vi "test Deployment With Configuration.vi"(8 "error in":errorcluster, 11 "TestCase in":refnum<class "Deployment.lvclass">) -> (0 "error out":errorcluster, 3 "TestCase out":refnum<class "Deployment.lvclass">)   [LabVIEW 2020, in "Deployment.lvclass"]
uses:
  Deployment.lvclass
  Shared/1553 Channel.ctl
  Shared/Terminal Name and Address.ctl
  Shared/Address.ctl
  Shared/Message Definition.ctl
  Shared/Message Type.ctl
  Shared/Terminal Endpoint.ctl
  Shared/Parameter Definition.ctl
  Deployment.lvclass/Deployment.ctl
  315b1c3a-44c8-49e8-b756-01f865c29b4a.vi
  <vilib>/addons/_JKI Toolkits/VI Tester/TestCase.llb/TestCase.lvclass
  niveristand-custom-device-testing-tools/VeriStandTestUtilities/VeriStandTestUtilities.lvlib
  Scripting/Ballard MIL-STD-1553 Scripting.lvlib
  C:/Program Files (x86)/National Instruments/LabVIEW 2020/vi.lib/addons/_JKI Toolkits/VI Tester/TestCase.llb/TestCase.lvclass
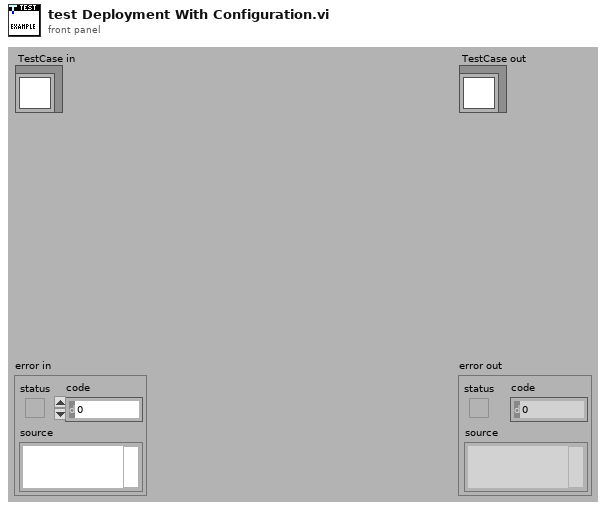
[diagram p1: front panel]
types:
  T1 = typedef "1553 Channel.ctl" = cluster{"HW channel":u16, "terminals":T2[], "messages":T4[], "acyclic frame names":string[]}
  T2 = typedef "Terminal Name and Address.ctl" = cluster{"name":string, "terminal address":T3}
  T3 = typedef "Address.ctl" = u16
  T4 = typedef "Message Definition.ctl" = cluster{"name":string, "message type":T5, "endpoint Rx":T6, "endpoint Tx":T6, "mode code":u16, "number of words":u16, "parameters":cluster{"name":string, "default value":dbl, "unit":string, "parameter definition":T7}[], "create timestamp channel":bool}
  T5 = typedef "Message Type.ctl" = string
  T6 = typedef "Terminal Endpoint.ctl" = cluster{"terminal address":T3, "subaddress":T3}
  T7 = typedef "Parameter Definition.ctl" = cluster{"start index":i32, "size (bits)":i32, "encoding":enum16{"BNR", "BCD", "Discrete"}, "signed":bool, "multiplier":dbl, "offset":dbl}
  T8 = typedef "Custom Device API.lvlib/Custom Device Item Ref.ctl" = u64
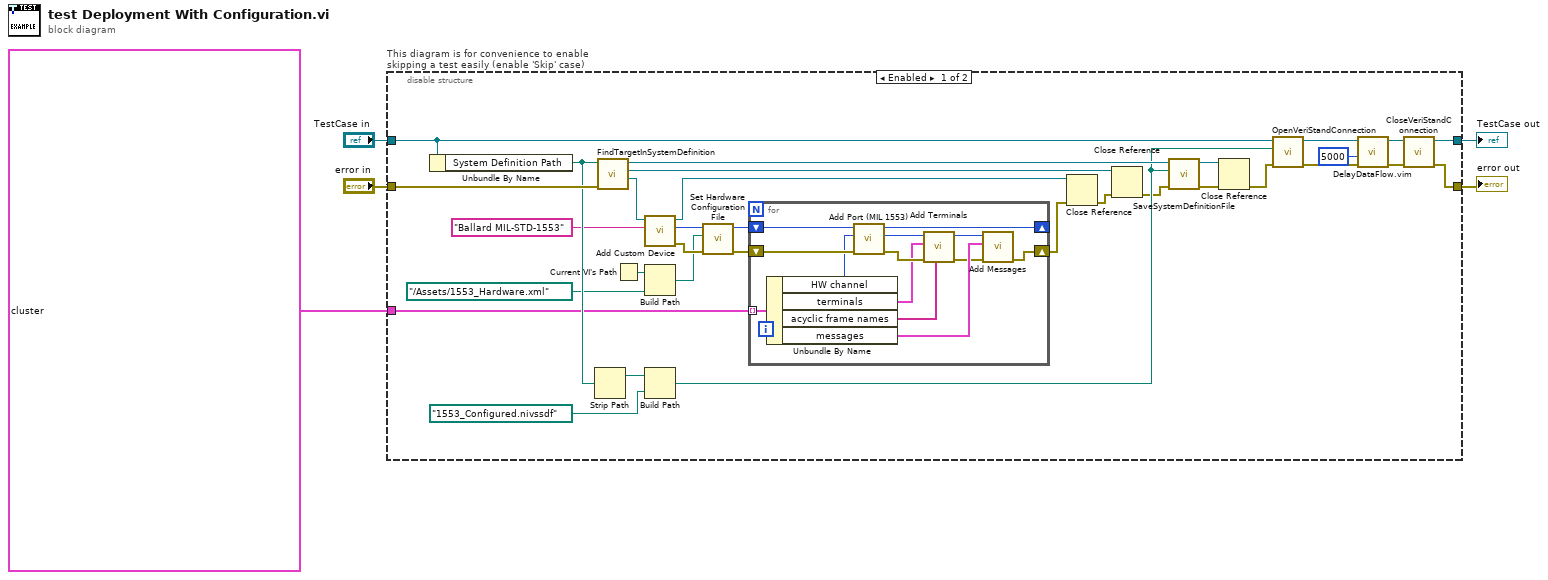
[diagram p0: block diagram]
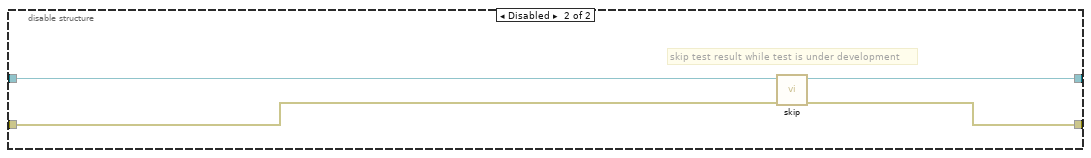
[diagram p2: hidden frame]
diagram:
  n1 = disable-structure "This diagram is for convenience to enable skipping a test easily (enable 'Skip' case)" shown="Enabled" {
    disable-tunnel: "TestCase in" -> [w30 w53]
    disable-tunnel: [w31 w51] -> w2
    disable-tunnel: [w33 w52] -> w4
    disable-tunnel: "error in" -> [w29 w50]
    disable-tunnel: T1[] [{"HW channel"=0, "terminals"=[{"name"="Bus Controller", "terminal address"=0}, {"name"="Remote Terminal 1", "terminal address"=1}, {"name"="Remote Terminal 15", "terminal address"=15}, {"name"="Remote Terminal 21", "terminal address"=21}, {"name"="Remote Terminal 31 (Broadcast)", "terminal address"=31}], "messages"=[{"name"="BC to RT 1.2", "message type"="BC to RT", "endpoint Rx"={"terminal address"=1, "subaddress"=2}, "endpoint Tx"={"terminal address"=0, "subaddress"=0}, "mode code"=0, "number of words"=3, "parameters"=[], "create timestamp channel"=FALSE}, {"name"="RT 31.15 to RT 21.21", "message type"="RT to RT", "endpoint Rx"={"terminal address"=31, "subaddress"=21}, "endpoint Tx"={"terminal address"=15, "subaddress"=21}, "mode code"=0, "number of words"=11, "parameters"=[], "create timestamp channel"=FALSE}, {"name"="BC to RT 3.0", "message type"="BC to RT", "endpoint Rx"={"terminal address"=1, "subaddress"=3}, "endpoint Tx"={"terminal address"=0, "subaddress"=0}, "mode code"=0, "number of words"=4, "parameters"=[], "create timestamp channel"=FALSE}, {"name"="RT 1.5 to BC", "message type"="RT to BC", "endpoint Rx"={"terminal address"=0, "subaddress"=0}, "endpoint Tx"={"terminal address"=1, "subaddress"=5}, "mode code"=0, "number of words"=6, "parameters"=[], "create timestamp channel"=FALSE}, {"name"="RT 1.6 to BC", "message type"="RT to BC", "endpoint Rx"={"terminal address"=0, "subaddress"=0}, "endpoint Tx"={"terminal address"=1, "subaddress"=6}, "mode code"=0, "number of words"=2, "parameters"=[], "create timestamp channel"=FALSE}, {"name"="RT 15.20 to RT 1.20", "message type"="RT to RT", "endpoint Rx"={"terminal address"=15, "subaddress"=20}, "endpoint Tx"={"terminal address"=1, "subaddress"=20}, "mode code"=0, "number of words"=4, "parameters"=[], "create timestamp channel"=FALSE}, {"name"="MC 16", "message type"="MC", "endpoint Rx"={"terminal address"=0, "subaddress"=0}, "endpoint Tx"={"terminal address"=1, "subaddress"=31}, "mode code"=16, "number of words"=1, "parameters"=[], "create timestamp channel"=FALSE}, {"name"="MC 17", "message type"="MC", "endpoint Rx"={"terminal address"=1, "subaddress"=31}, "endpoint Tx"={"terminal address"=0, "subaddress"=0}, "mode code"=17, "number of words"=1, "parameters"=[], "create timestamp channel"=FALSE}, {"name"="BC to RT 31.28", "message type"="BC to RT", "endpoint Rx"={"terminal address"=31, "subaddress"=28}, "endpoint Tx"={"terminal address"=0, "subaddress"=0}, "mode code"=0, "number of words"=6, "parameters"=[], "create timestamp channel"=FALSE}, {"name"="MC 1", "message type"="MC", "endpoint Rx"={"terminal address"=31, "subaddress"=31}, "endpoint Tx"={"terminal address"=0, "subaddress"=0}, "mode code"=1, "number of words"=0, "parameters"=[], "create timestamp channel"=FALSE}], "acyclic frame names"=["acyclicFrame ID56"]}] -> [w13 _]
    frame Enabled {
      n2 = Unbundle By Name(w30) -> ("System Definition Path"=w27:path)
      n3 = Strip Path(path=w27) -> (stripped path=w26:path)  [unwired: 1 out]
      n4 = call "FindTargetInSystemDefinition.vi"("error in"=w29, "system definition path"=w27) -> ("Target"=w24:refnum<k24>, "Root"=w19:refnum<k24>, "System Definition"=w28:refnum<k24>)  [unwired: 6 in, 1 out]
      n5 = Current VI's Path() -> (path=w8:path)
      n6 = call "Add Custom Device.vi"("name"="Ballard MIL-STD-1553", "target in"=w24) -> ("error out"=w11:errorcluster, "Ballard MIL-STD-1553 custom device"=w12:T8, "target out"=w17:refnum<k24>)  [unwired: 7 in]
      n7 = Build Path(base path=w8, name or relative path=path "../Assets/1553_Hardware.xml") -> (appended path=w6:path)
      n8 = Build Path(base path=w26, name or relative path=path "1553_Configured.nivssdf") -> (appended path=w20:path)
      n9 = call "Set Hardware Configuration File.vi"("error in"=w11, "hardware configuration file path"=w6, "Ballard MIL-STD 1553 custom device in"=w12) -> ("error out"=w10:errorcluster, "Ballard MIL-STD 1553 custom device out"=w9:T8)  [unwired: 7 in]
      n10 = for {
        shift-right: [w45] -> _
        shift-left: w9 -> [w48]
        tunnel: w13 -> [w49] mode=indexing
        shift-right: [w43] -> w15
        shift-left: w10 -> [w47]
        n11 = Unbundle By Name(w49) -> ("HW channel"=w46:u16, "terminals"=w38:T2[], "acyclic frame names"=w37:string[], "messages"=w44:T4[])
        n12 = call "Add Port (MIL 1553).vi"("error in"=w47, "port number"=w46, "Ballard MIL-STD 1553 custom device in"=w48) -> ("error out"=w41:errorcluster, "port"=w42:T8, "Ballard MIL-STD 1553 custom device out"=w45:T8)  [unwired: 6 in]
        n13 = call "Add Terminals.vi"("acyclic frame names"=w37, "error in"=w41, "terminals"=w38, "port in"=w42) -> ("error out"=w39:errorcluster, "port out"=w40:T8)  [unwired: 6 in]
        n14 = call "Add Messages.vi"("error in"=w39, "messages"=w44, "port in"=w40) -> ("error out"=w43:errorcluster)  [unwired: 7 in, 1 out]
      }
      n15 = Close Reference(reference=w17, error in (no error)=w15) -> (error out=w16:errorcluster)
      n16 = Close Reference(reference=w19, error in (no error)=w16) -> (error out=w18:errorcluster)
      n17 = call "SaveSystemDefinitionFile.vi"("error in (no error)"=w18, "System Definition File in"=w20, "System Definition Reference in"=w28) -> ("error out"=w22:errorcluster, "System Definition Reference out"=w23:refnum<k24>)  [unwired: 7 in]
      n18 = Close Reference(reference=w23, error in (no error)=w22) -> (error out=w21:errorcluster)
      n19 = call-dynamic "OpenVeriStandConnection.vi"("error in (no error)"=w21, "System Definition File"=w20, "VeriStand Test Case in"=w30) -> ("error out"=w36:errorcluster, "VeriStand Test Case out"=w32:refnum<class "Deployment.lvclass">)  [unwired: 6 in, 1 out]
      n20 = call "DelayDataFlow.vim"("value in"=w36, "milliseconds to wait"=u32 5000) -> ("value out"=w34:errorcluster)  [unwired: 2 in, 1 out]
      n21 = call-dynamic "CloseVeriStandConnection.vi"("error in (no error)"=w34, "VeriStand Test Case in"=w32) -> ("error out"=w33:errorcluster, "VeriStand Test Case out"=w31:refnum<class "Deployment.lvclass">)  [unwired: 8 in]
    }
    frame Disabled {
      # "skip test result while test is under development"
      n22 = call <vilib>:"skip.vi"("error in (no error)"=w50, "TestCase in"=w53) -> ("error out"=w52:errorcluster, "TestCase out"=w51:refnum<class "Deployment.lvclass">)  [unwired: 8 in]
    }
  }
  "error out" <- w4
  "TestCase out" <- w2
